vi "Enable Serial Input Channels.vi"(0 "fpga interface in":refnum<k20>, 5 "serial input channels":string[](array[string]), 11 "error in (no error)":errorcluster) -> (4 "fpga interface out":refnum<k20>, 15 "error out":errorcluster)   [LabVIEW 2023, in "GettingStarted_Acq_148X_Host.lvlib"]
uses:
  GettingStarted_Acq_148X_Host.lvlib
  Types/148x_Acq_FPGA_Reference.ctl
  <instrlib>/FlexRIO/API/Host/v1/NI FlexRIO/API/Get Property Reference - Fpga Small.vi
  <vilib>/Utility/error.llb/Error Cluster From Error Code.vi
  <vilib>/rvi/errors/niLvFpgaAdjustHostInterfaceError.vi
  <vilib>/rvi/interface/nirviReadWriteControl/nirviReadWriteControl.xnode
  <resource>/objmgr/niflexrioapi.rc
  <instrlib>/FlexRIO/API/Host/v1/NI FlexRIO API v1.lvlib
  NiFpgaLv.dll
  <vilib>/rvi/interface/Simulation/niFpgaSimulationCallBeginRW.vi
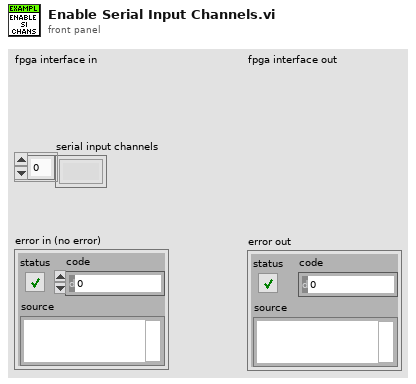
[diagram p1: front panel]
types:
  T1 = typedef "GettingStarted_Acq_148X_Host.lvlib/148x_Acq_FPGA_Reference.ctl" = refnum<k20>
  T2 = cluster{"channel acq config":cluster{"stop timeout (cycles)":u32, "first packet data type select mask":u64, "last packet data type select mask":u64, "first and last packet virtual channel must match":bool}, "virtual channel packet filter mask":u16, "data type packet filter mask":u64, "select corrected csi-2 data":bool, "enable channel":bool}[]
  T3 = cluster{"channel acq config":cluster{"stop timeout (cycles)":u32, "first packet data type select mask":u64, "last packet data type select mask":u64, "first and last packet virtual channel must match":bool}, "virtual channel packet filter mask":u16, "data type packet filter mask":u64, "select corrected csi-2 data":bool, "enable channel":bool}
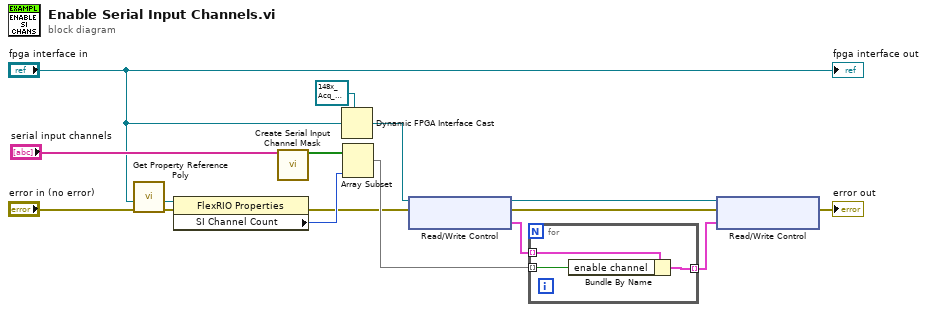
[diagram p0: block diagram]
diagram:
  n1 = call-poly <instrlib>:"Get Property Reference Poly.vi"("error in (no error)"="error in (no error)", "fpga interface in"="fpga interface in") -> ("error out"=w13:errorcluster, "property reference"=w14:refnum<k20>)  [unwired: 4 in, 1 out]
  n2 = property class="FlexRIO Properties"(reference=w14, error in=w13) -> (error out=w5:errorcluster, "SI Channel Count"=w8:i32)  [unwired: 1 out]
  n3 = call "Create Serial Input Channel Mask.vi"("serial channels"="serial input channels") -> ("serial input channel mask"=w10:bool[])  [unwired: 14 in]
  n4 = Dynamic FPGA Interface Cast(Session In=T1 refnum ("FPGA VI Reference Out"), Type="fpga interface in") -> (Session Out=w3:T1)
  n5 = Array Subset(array=w10, length=w8) -> (w6:bool[])  [unwired: 1 in]
  n6 = xnode "Read/Write Control"("FPGA VI Reference In"=w3, "error in"=w5) -> ("FPGA VI Reference Out"=w2:T1, "error out"=w4:errorcluster, "channel configs"=w7:T2)
  n7 = for {
    tunnel: w7 -> [w19] mode=indexing
    tunnel: w6 -> [w18] mode=indexing
    tunnel: [w17] -> w1 mode=indexing
    n8 = Bundle By Name(cluster=w19, "enable channel"=w18) -> (w17:T3)
  }
  n9 = xnode "Read/Write Control"("FPGA VI Reference In"=w2, "error in"=w4, "channel configs"=w1) -> ("error out"=→"error out":errorcluster)  [unwired: 1 out]
  "fpga interface out" <- "fpga interface in"
